vi "FTW-TestExecutiveGUI-Core_Process.vi"(0 "FTW Actor Instance Configuration":string="{\n  \"Identity\": \"ActorName\",\n  \"InboxAddress\": \"inproc://*\",\n  \"LoggerAddress\": \"\",\n  \"DebugEnableInboxLogging\": false,\n  \"DebugEnableJobLogging\": false,\n  \"LauncherAddress\": \"\",\n  \"Connections\": {\n    \"ConnectionOne\": \"inproc://connection-one\",\n    \"ConnectionTwo\": \"tcp://localhost/connection-two\"\n  },\n  \"Publishers\": {\n    \"PublisherOne\": \"inproc://publisher-one\",\n    \"PublisherTwo\": \"tcp://localhost/publisher-two\"\n  },\n  \"Subscriptions\": {\n    \"SubscriptionOne\": \"inproc://subscription-one\",\n    \"SubscriptionTwo\": \"tcp://localhost/subscription-two\"\n  },\n  \"My Data\": false,\n  \"Refresh Period\": 2\n}", 11 "ErrorIn":errorcluster) -> (15 "Error":errorcluster)   [LabVIEW 2015, in "FTW-TestExecutiveGUI-Core.lvclass"]
uses:
  FTW-TestExecutiveGUI-Core.lvclass
  FTW-TestExecutiveGUI-Core.lvclass/FTW-TestExecutiveGUI-Core.ctl
  source/actor/Instance/FTW-ActorInstance.lvclass/FTW-ActorInstance.ctl
  source/actor/JobSequencer/FTW-SEQ-Current.vi
  source/actor/Message/Base/FTW-Message.lvclass
  source/actor/Instance/FTW-ActorInstance.lvclass
  source/actor/Message/Request/FTW-Message-IncomingRequest.lvclass
  source/actor/Instance-Extended/FTW-ActorExtended.lvclass
panel:
  # "#TODO\nhide controls for a GUI"
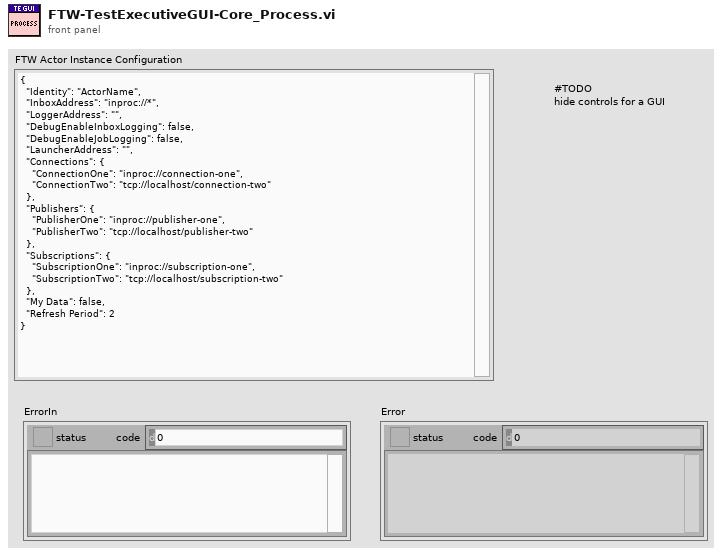
[diagram p1: front panel]
types:
  T1 = cluster{"Incoming Requests":refnum<event-registration>, "Local Messages":refnum<event-registration>, "Subscriber Registration":refnum<event-registration>}
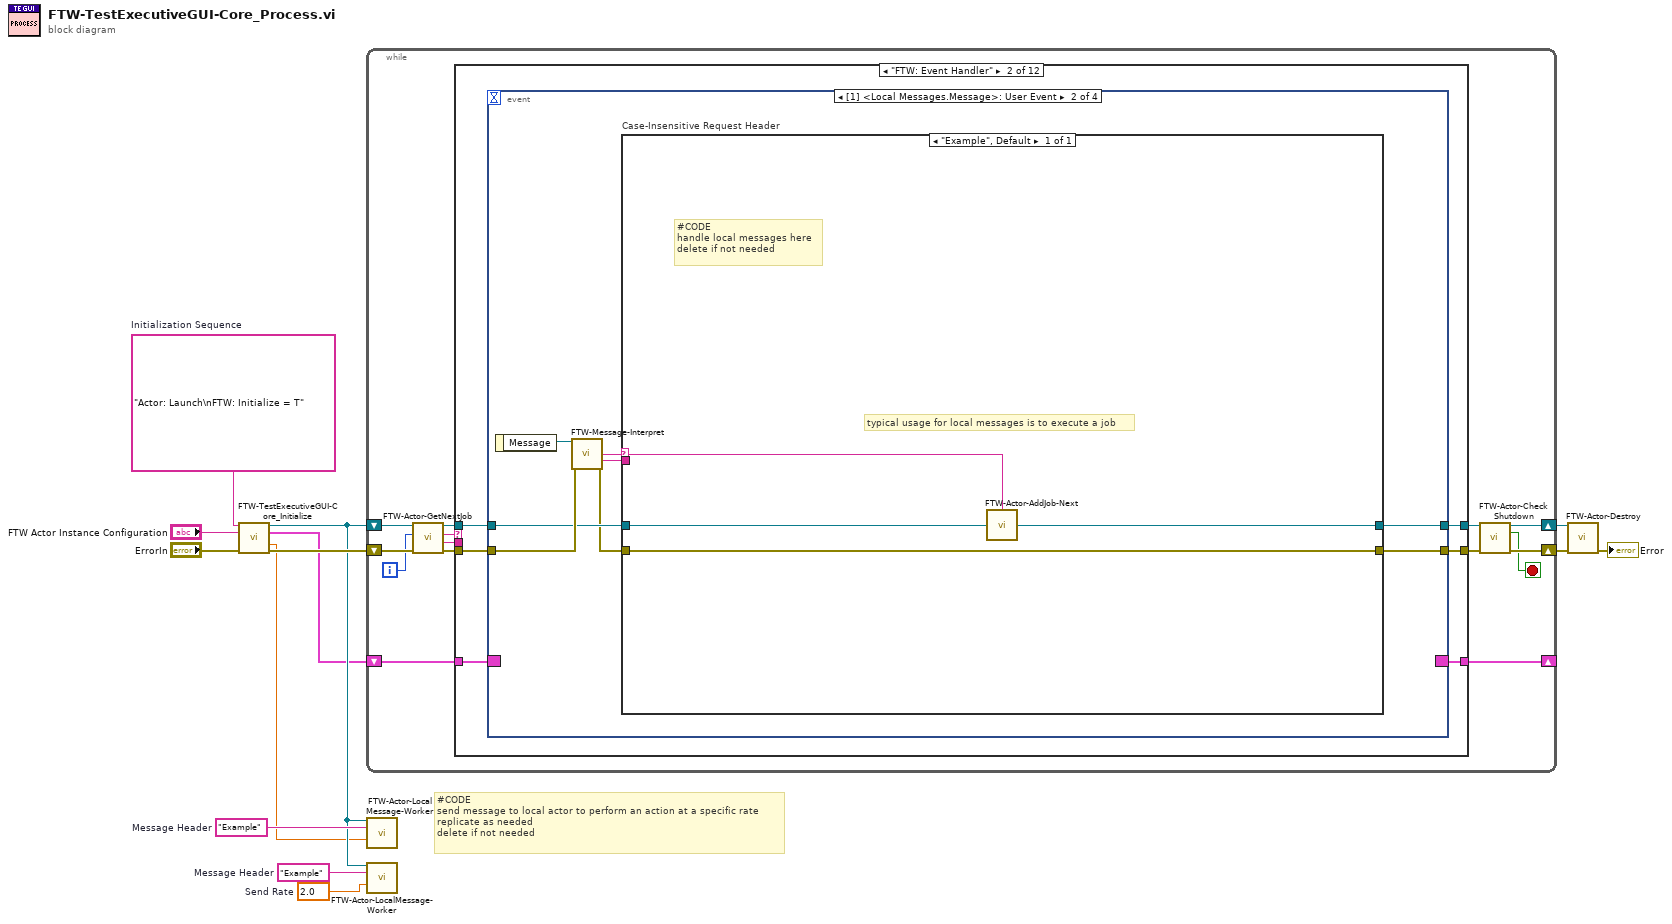
[diagram p0: block diagram]
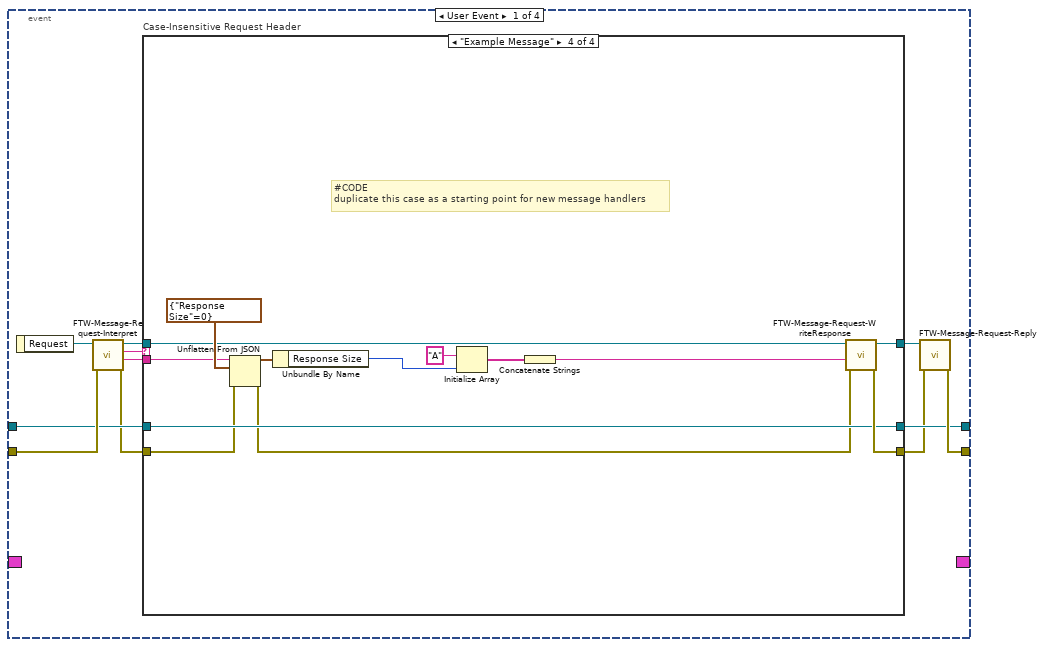
[diagram p3: hidden frame]
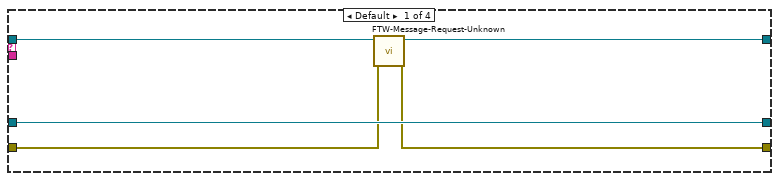
[diagram p4: hidden frame]
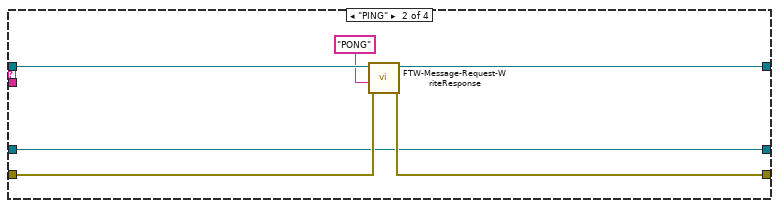
[diagram p5: hidden frame]
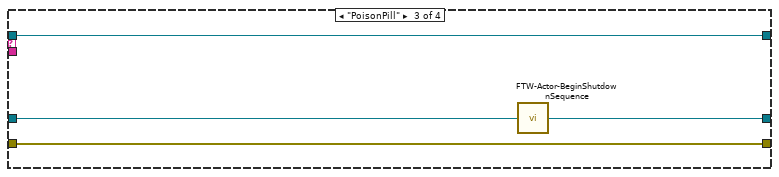
[diagram p6: hidden frame]
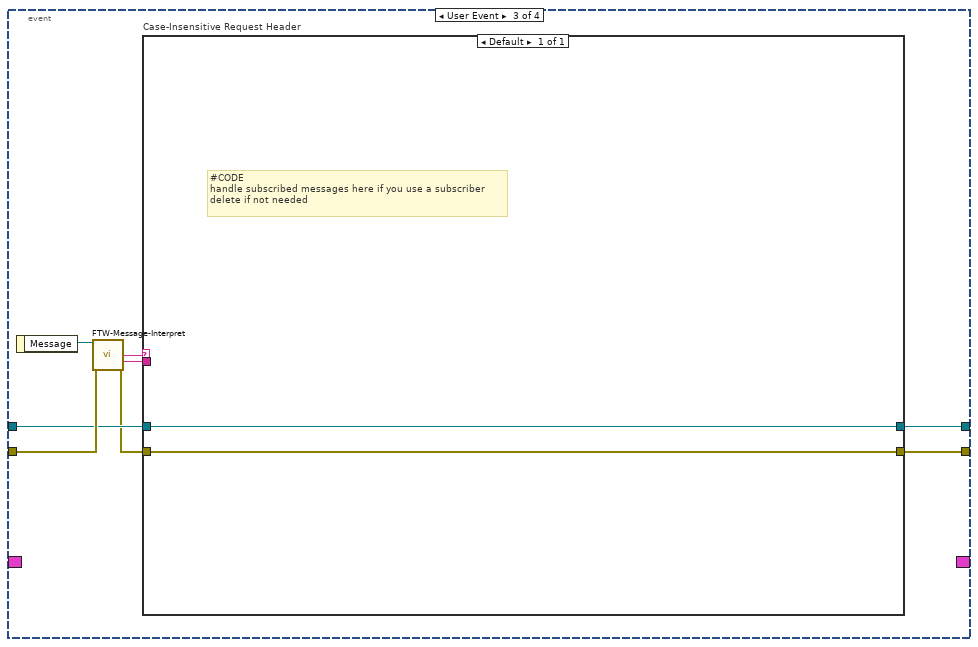
[diagram p7: hidden frame]
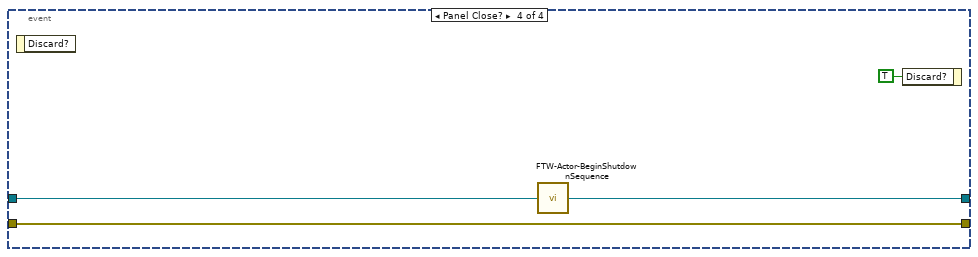
[diagram p8: hidden frame]
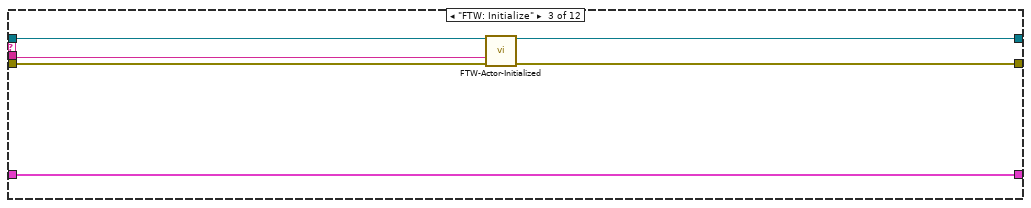
[diagram p9: hidden frame]
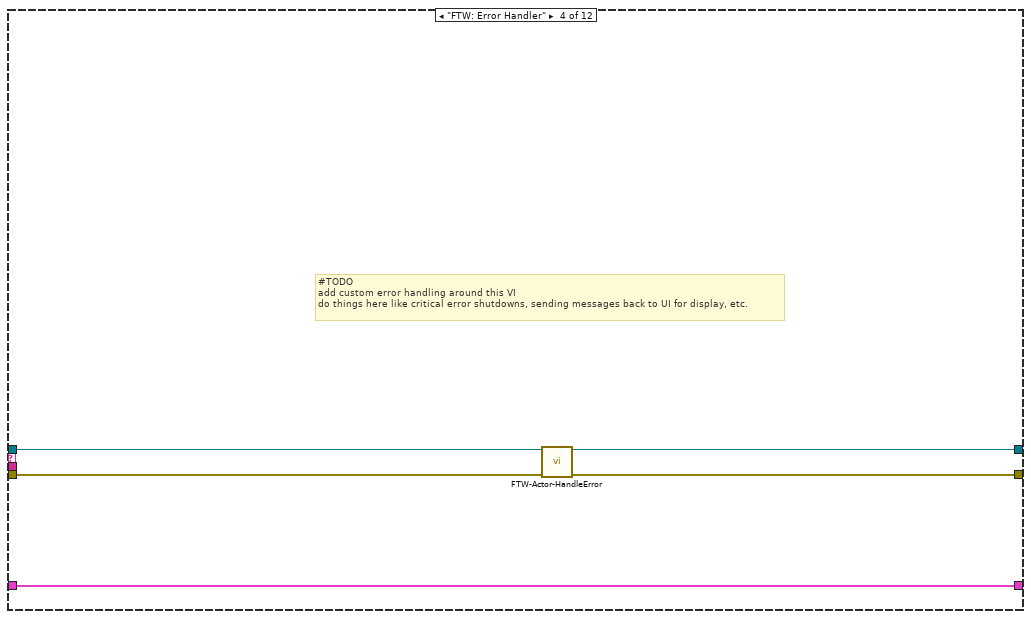
[diagram p10: hidden frame]
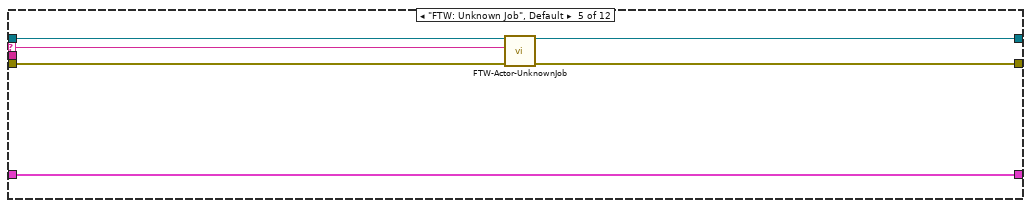
[diagram p11: hidden frame]
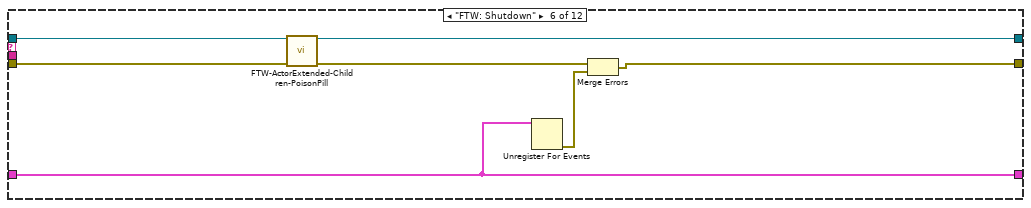
[diagram p12: hidden frame]
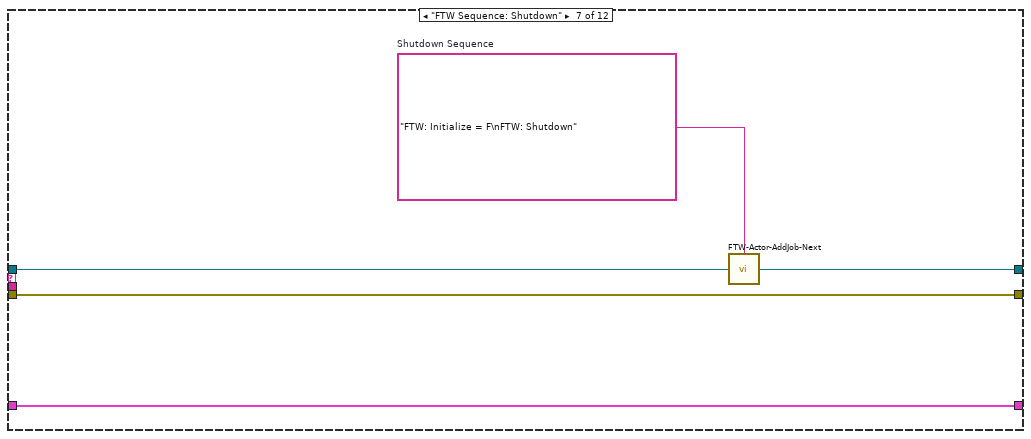
[diagram p13: hidden frame]
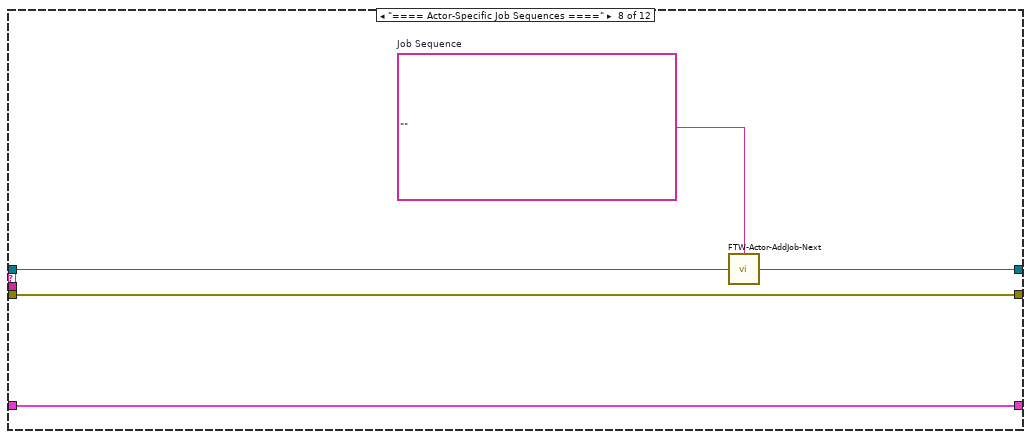
[diagram p14: hidden frame]
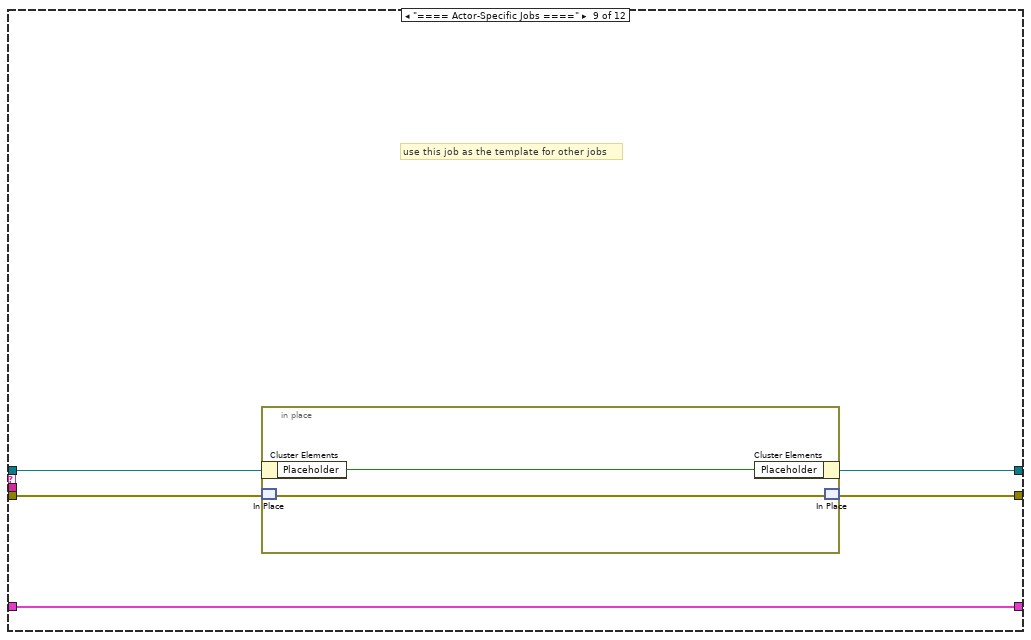
[diagram p15: hidden frame]
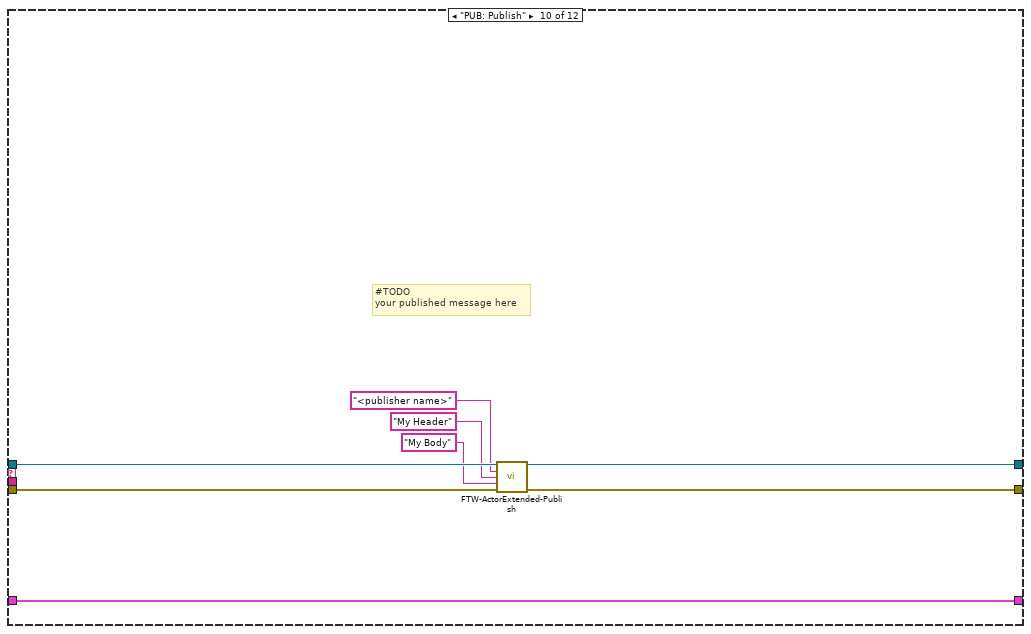
[diagram p16: hidden frame]
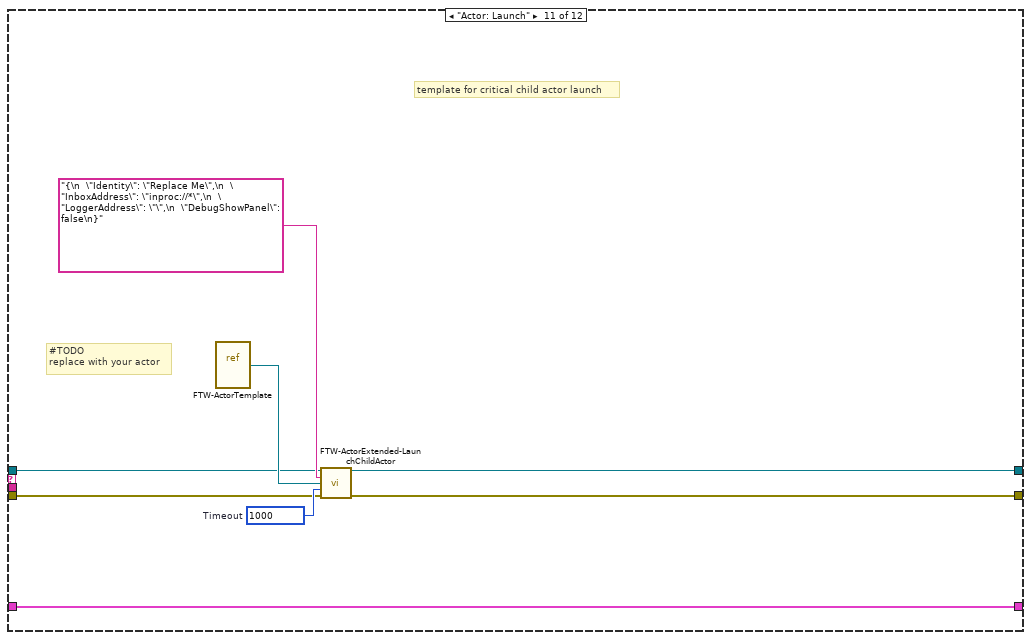
[diagram p17: hidden frame]
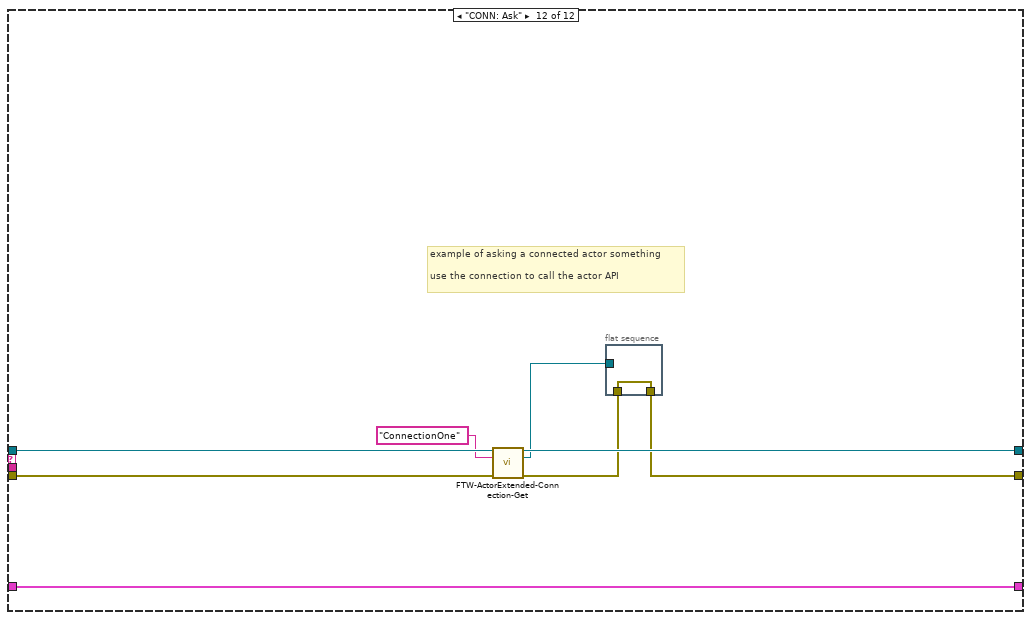
[diagram p18: hidden frame]
diagram:
  w5 = 2.0  # Send Rate
  w4 = "Example"  # Message Header
  w6 = "Example"  # Message Header
  w9 = "Actor: Launch\nFTW: Initialize = T"  # Initialization Sequence
  # "#CODE\nsend message to local actor to perform an action at a specific rate\nreplicate as needed\ndelete if not needed"
  n1 = call "FTW-TestExecutiveGUI-Core_Initialize.vi"("Initialization Sequence"=w9, "FTW Actor Instance Configuration"="FTW Actor Instance Configuration", "error in (no error)"="ErrorIn") -> ("Actor Template-Core out"=w3:refnum<class "FTW-TestExecutiveGUI-Core.lvclass">, "Event Refnums"=w1:T1, "Refresh Period"=w2:dbl, "error out"=w10:errorcluster)  [unwired: 9 in]
  n2 = while {
    shift-right: [w17] -> w12
    shift-left: w10 -> [w24]
    shift-right: [w14] -> _
    shift-left: w1 -> [w27]
    shift-right: [w19] -> w13
    shift-left: w3 -> [w26]
    i -> [w15]
    stop <- w16 stop-if-true
    n3 = call "FTW-Actor-GetNextJob.vi"("error in"=w24, "Jobs Performed"=w15, "FTW Actor Instance"=w26) -> ("error out"=w23:errorcluster, "Job Data"=w21:string, "Job Name"=w22:string, "FTW Actor Instance out"=w25:refnum<class "FTW-TestExecutiveGUI-Core.lvclass">)  [unwired: 5 in]
    n4 = case shown="\"FTW: Event Handler\"" w22 {
      selector: w22 -> [_ _ _ _ w113 _ _ _ _ _ _ _]
      tunnel: [w29 w36 w104 w108 w116 w124 w129 w134 w138 w148 w153 w159] -> w18
      tunnel: w23 -> [w29 w35 w106 w110 w117 w125 w129 w134 w139 w149 w154 w165]
      tunnel: w27 -> [w30 w31 w107 w112 w118 w122 w130 w135 w140 w150 w158 w166]
      tunnel: [w30 w34 w107 w112 w118 w122 w130 w135 w140 w150 w158 w166] -> w14
      tunnel: w21 -> [_ _ w102 _ _ _ _ _ _ _ _ _]
      tunnel: [w28 w33 w105 w109 w114 w119 w127 w132 w136 w146 w151 w163] -> w20
      tunnel: w25 -> [w28 w32 w103 w111 w115 w120 w128 w133 w137 w147 w152 w164]
      frame "==== Featherweight Framework Jobs ====" {
      }
      frame "FTW: Event Handler" {
        n5 = event shown="[1] <Local Messages.Message>: User Event" {
          selector: w31 -> [_ _ _ _]
          dyn-events: [_ _ _ _] -> w34
          timeout: _ -> [_ _ _ _]
          tunnel: [w46 w78 w90 w100] -> w36
          tunnel: w35 -> [w45 w82 w94 w100]
          tunnel: [w40 w79 w91 w98] -> w33
          tunnel: w32 -> [w44 w81 w93 w99]
          event User Event {
            n6 = event-data() -> ("Request"=w47:refnum<class "FTW-Message-IncomingRequest.lvclass">)  [unwired: 1 in]
            n7 = call "FTW-Message-Request-Interpret.vi"("error in"=w45, "FTW Incoming Request"=w47) -> ("error out"=w43:errorcluster, "Request Body"=w37:string, "Request Header"=w41:string, "FTW Incoming Request out"=w42:refnum<class "FTW-Message-IncomingRequest.lvclass">)  [unwired: 6 in]
            n8 = case "Case-Insensitive Request Header" shown="\"Example Message\"" w41 {
              tunnel: [w50 w56 w61 w75] -> w39
              tunnel: w43 -> [w51 w57 w61 w64]
              tunnel: [w52 w55 w62 w73] -> w40
              tunnel: w44 -> [w52 w55 w60 w73]
              tunnel: w42 -> [w49 w58 w59 w65]
              tunnel: [w48 w54 w59 w74] -> w38
              tunnel: w37 -> [_ _ _ w63]
              frame Default {
                n9 = call "FTW-Message-Request-Unknown.vi"("error in"=w51, "FTW Incoming Request"=w49) -> ("error out"=w50:errorcluster, "FTW Incoming Request Out"=w48:refnum<class "FTW-Message-IncomingRequest.lvclass">)  [unwired: 8 in]
              }
              frame "PING" {
                n10 = call "FTW-Message-Request-WriteResponse.vi"("error in"=w57, "Response Body"="PONG" ("Response Header"), "FTW Incoming Request"=w58) -> ("error out"=w56:errorcluster, "FTW Incoming Request out"=w54:refnum<class "FTW-Message-IncomingRequest.lvclass">)  [unwired: 7 in]
              }
              frame "PoisonPill" {
                n11 = call "FTW-Actor-BeginShutdownSequence.vi"("FTW Actor Instance"=w60) -> ("FTW Actor Instance out"=w62:refnum<class "FTW-TestExecutiveGUI-Core.lvclass">)  [unwired: 3 in]
              }
              frame "Example Message" {
                # "#CODE\nduplicate this case as a starting point for new message handlers"
                n12 = Unflatten From JSON(JSON string=w63, type and defaults=cluster{"Response Size":i32} {"Response Size"=0}, error in (no error)=w64) -> (value=w70:cluster{"Response Size":i32}, error out=w72:errorcluster)  [unwired: 4 in]
                n13 = Unbundle By Name(w70) -> ("Response Size"=w69:i32)
                n14 = Initialize Array("A", w69) -> (w67:string[])
                n15 = Concatenate Strings(w67) -> (w66:string)
                n16 = call "FTW-Message-Request-WriteResponse.vi"("error in"=w72, "Response Body"=w66, "FTW Incoming Request"=w65) -> ("error out"=w75:errorcluster, "FTW Incoming Request out"=w74:refnum<class "FTW-Message-IncomingRequest.lvclass">)  [unwired: 7 in]
              }
            }
            n17 = call "FTW-Message-Request-Reply.vi"("FTW: Reply Error"=w39, "FTW Incoming Request"=w38) -> ("error out"=w46:errorcluster)  [unwired: 8 in, 1 out]
          }
          event User Event {
            n18 = event-data() -> ("Message"=w83:refnum<class "FTW-Message.lvclass">)  [unwired: 1 in]
            n19 = call-dynamic "FTW-Message-Interpret.vi"("FTW Message"=w83, "error in"=w82) -> ("Message Header"=w77:string, "Message Body"=w76:string, "error out"=w80:errorcluster)  [unwired: 9 in, 2 out]
            n20 = case "Case-Insensitive Request Header" shown="\"Example\", Default" w77 {
              selector: w77 -> [w84]
              tunnel: [w86] -> w78
              tunnel: w80 -> [w86]
              tunnel: [w85] -> w79
              tunnel: w81 -> [w87]
              tunnel: w76 -> [_]
              frame "Example", Default {
                # "#CODE\nhandle local messages here\ndelete if not needed"
                # "typical usage for local messages is to execute a job"
                n21 = call "FTW-Actor-AddJob-Next.vi"("Add Next in Job Queue"=w84, "FTW Actor Instance"=w87) -> ("FTW Actor Instance out"=w85:refnum<class "FTW-TestExecutiveGUI-Core.lvclass">)  [unwired: 2 in]
              }
            }
          }
          event User Event {
            n22 = event-data() -> ("Message"=w95:refnum<class "FTW-Message.lvclass">)  [unwired: 1 in]
            n23 = call-dynamic "FTW-Message-Interpret.vi"("FTW Message"=w95, "error in"=w94) -> ("Message Header"=w89:string, "Message Body"=w88:string, "error out"=w92:errorcluster)  [unwired: 9 in, 2 out]
            n24 = case "Case-Insensitive Request Header" shown="Default" w89 {
              tunnel: [w96] -> w90
              tunnel: w92 -> [w96]
              tunnel: [w97] -> w91
              tunnel: w93 -> [w97]
              tunnel: w88 -> [_]
              frame Default {
                # "#CODE\nhandle subscribed messages here if you use a subscriber\ndelete if not needed"
              }
            }
          }
          event Panel Close? {
            n25 = event-data() -> ()  [unwired: 1 in, 1 out]
            n26 = call "FTW-Actor-BeginShutdownSequence.vi"("FTW Actor Instance"=w99) -> ("FTW Actor Instance out"=w98:refnum<class "FTW-TestExecutiveGUI-Core.lvclass">)  [unwired: 3 in]
            n27 = event-data("Discard?"=TRUE) -> ()  [unwired: 1 in, 1 out]
          }
        }
      }
      frame "FTW: Initialize" {
        n28 = call-dynamic "FTW-Actor-Initialized.vi"("FTW Actor Instance"=w103, "Positive Init?"=w102, "error in"=w106) -> ("FTW Actor Instance out"=w105:refnum<class "FTW-TestExecutiveGUI-Core.lvclass">, "error out"=w104:errorcluster)  [unwired: 11 in]
      }
      frame "FTW: Error Handler" {
        # "#TODO\nadd custom error handling around this VI\ndo things here like critical error shutdowns, sending messages back to UI for display, etc."
        n29 = call-dynamic "FTW-Actor-HandleError.vi"("FTW Actor Instance"=w111, "error in"=w110) -> ("FTW Actor Instance out"=w109:refnum<class "FTW-TestExecutiveGUI-Core.lvclass">, "error out"=w108:errorcluster)  [unwired: 10 in, 2 out]
      }
      frame "FTW: Unknown Job", Default {
        n30 = call-dynamic "FTW-Actor-UnknownJob.vi"("FTW Actor Instance"=w115, "Unknown Job"=w113, "error in"=w117) -> ("FTW Actor Instance out"=w114:refnum<class "FTW-TestExecutiveGUI-Core.lvclass">, "error out"=w116:errorcluster)  [unwired: 11 in]
      }
      frame "FTW: Shutdown" {
        n31 = call "FTW-ActorExtended-Children-PoisonPill.vi"("FTW-ActorExtended In"=w120, "error in"=w125) -> ("FTW-ActorExtended Out"=w119:refnum<class "FTW-TestExecutiveGUI-Core.lvclass">, "error out"=w121:errorcluster)  [unwired: 12 in]
        n32 = Unregister For Events(event registration refnum=w122) -> (error out=w123:errorcluster)  [unwired: 1 in]
        n33 = Merge Errors(w121, w123) -> (w124:errorcluster)
      }
      frame "FTW Sequence: Shutdown" {
        w126 = "FTW: Initialize = F\nFTW: Shutdown"  # Shutdown Sequence
        n34 = call "FTW-Actor-AddJob-Next.vi"("Add Next in Job Queue"=w126, "FTW Actor Instance"=w128) -> ("FTW Actor Instance out"=w127:refnum<class "FTW-TestExecutiveGUI-Core.lvclass">)  [unwired: 2 in]
      }
      frame "==== Actor-Specific Job Sequences ====" {
        w131 = ""  # Job Sequence
        n35 = call "FTW-Actor-AddJob-Next.vi"("Add Next in Job Queue"=w131, "FTW Actor Instance"=w133) -> ("FTW Actor Instance out"=w132:refnum<class "FTW-TestExecutiveGUI-Core.lvclass">)  [unwired: 2 in]
      }
      frame "==== Actor-Specific Jobs ====" {
        # "use this job as the template for other jobs"
        n36 = in-place {
          n37 = in-place-cluster #1(w137) -> ("Placeholder"=w141:bool)
          n38 = in-place-match #2(w139) -> (w142:errorcluster)
          n39 = in-place-cluster #1("Placeholder"=w141) -> (w136:refnum<class "FTW-TestExecutiveGUI-Core.lvclass">)
          n40 = in-place-match #2(w142) -> (w138:errorcluster)
        }
      }
      frame "PUB: Publish" {
        # "#TODO\nyour published message here"
        n41 = call "FTW-ActorExtended-Publish.vi"("FTW-ActorExtended In"=w147, "Publisher Name"="<publisher name>", "Message Header"="My Header" ("Header"), "Message Body"="My Body" ("Header"), "error in"=w149) -> ("FTW-ActorExtended Out"=w146:refnum<class "FTW-TestExecutiveGUI-Core.lvclass">, "error out"=w148:errorcluster)  [unwired: 9 in]
      }
      frame "Actor: Launch" {
        w157 = 1000  # Timeout
        # "#TODO\nreplace with your actor"
        # "template for critical child actor launch"
        n42 = vi-ref "FTW-ActorTemplate.vi"() -> (w156:refnum<vi>)
        n43 = call "FTW-ActorExtended-LaunchChildActor.vi"("FTW Actor Connector Type"=w152, "Configuration"="{\n  \"Identity\": \"Replace Me\",\n  \"InboxAddress\": \"inproc://*\",\n  \"LoggerAddress\": \"\",\n  \"DebugShowPanel\": false\n}", "Actor VI Refnum"=w156, "Timeout"=w157, "error in"=w154) -> ("FTW-ActorExtended.lvclass"=w151:refnum<class "FTW-TestExecutiveGUI-Core.lvclass">, "error out"=w153:errorcluster)  [unwired: 6 in, 3 out]
      }
      frame "CONN: Ask" {
        # "example of asking a connected actor something\n\nuse the connection to call the actor API"
        n44 = call "FTW-ActorExtended-Connection-Get.vi"("FTW-ActorExtended In"=w164, "Connector Name"="ConnectionOne" ("Publisher Name"), "error in"=w165) -> ("FTW-ActorExtended Out"=w163:refnum<class "FTW-TestExecutiveGUI-Core.lvclass">, "FTW Actor Connector"=w161:refnum<class "FTW-ActorConnector.lvclass">, "error out"=w160:errorcluster)  [unwired: 10 in]
        n45 = flat-sequence {
          tunnel: w161 -> [_]
          tunnel: w160 -> [w167]
          tunnel: [w167] -> w159
          frame #0 {
          }
        }
      }
    }
    n46 = call "FTW-Actor-CheckShutdown.vi"("FTW Actor Instance"=w20, "error in"=w18) -> ("FTW Actor Instance out"=w19:refnum<class "FTW-TestExecutiveGUI-Core.lvclass">, "Shutdown?"=w16:bool, "error out"=w17:errorcluster)  [unwired: 11 in]
  }
  n47 = call-dynamic "FTW-Actor-LocalMessage-Worker.vi"("FTW-ActorInstance In"=w3, "Message Header"=w6, "Send Rate"=w2) -> ()  [unwired: 13 in]
  n48 = call-dynamic "FTW-Actor-LocalMessage-Worker.vi"("FTW-ActorInstance In"=w3, "Message Header"=w4, "Send Rate"=w5) -> ()  [unwired: 13 in]
  n49 = call-dynamic "FTW-Actor-Destroy.vi"("FTW Actor Instance"=w13, "error in"=w12) -> ("error out"=→"Error":errorcluster)  [unwired: 13 in]
